vi "Fetch Trace (Reflection Measurement).vi"(8 "error in (no error)":errorcluster, 9 "Timeout (10000ms)":i32=10000, 10 "Data Type (0: Data)":i32(ring) items=["Data", "Memory"], 11 "VISA resource name":refnum<visa-resource-name>) -> (0 "error out":errorcluster, 2 "Trace Data":dbl[](array[numeric]), 3 "VISA resource name out":refnum<visa-resource-name>)   [LabVIEW 2022 SP3, in "Agilent N934X Series.lvlib"]
doc: "Fetches trace of Reflection Measurement from the spectrum analyzer and does not initiate data acquisition.\n\nNote:\n\nThis VI does not check the instrument status. Typically, you call this VI only in a sequence of calls to other low-level instrument driver VIs. The sequence performs one operation. You use the low-level VIs to optimize one or more aspects of interaction with the instrument. If you want to check the instrument status, call the <B>Error Query VI</B> at the conclusion of the sequence.\n\nThis VI is only applicable for N9321C, N9322C, N9323C, N9324C models."
uses:
  <instrlib>/Agilent N934X Series/Agilent N934X Series.lvlib
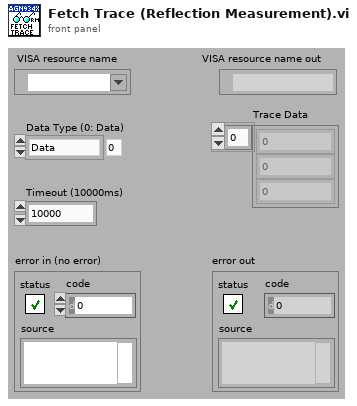
[diagram p1: front panel]
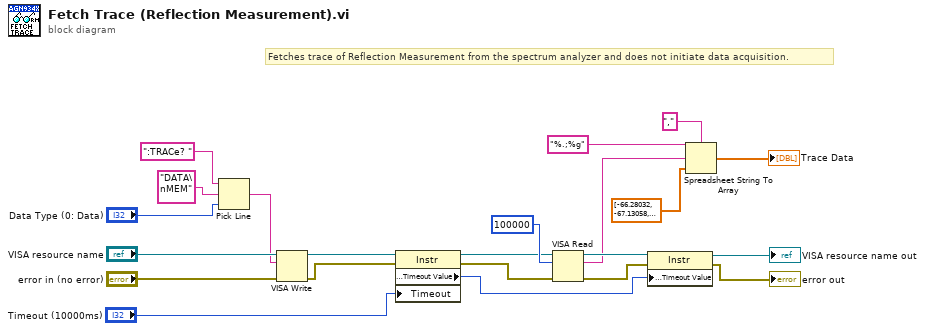
[diagram p0: block diagram]
diagram:
  # "Fetches trace of Reflection Measurement from the spectrum analyzer and does not initiate data acquisition."
  n1 = Pick Line(string ("")=":TRACe? ", multi-line string="DATA\nMEM", line index="Data Type (0: Data)") -> (output string=w2:string)
  n2 = VISA Write(VISA resource name="VISA resource name", write buffer=w2, error in (no error)="error in (no error)") -> (VISA resource name out=w19:refnum<visa-resource-name>, error out=w18:errorcluster)  [unwired: 1 out]
  n3 = property class="Instr"(reference=w19, error in=w18, "Timeout"="Timeout (10000ms)") -> (reference out=w17:refnum<visa-resource-name>, error out=w16:errorcluster, "General Settings:Timeout Value"=w14:u32)
  n4 = VISA Read(VISA resource name=w17, byte count=u32 100000, error in (no error)=w16) -> (VISA resource name out=w13:refnum<visa-resource-name>, read buffer=w11:string, error out=w12:errorcluster)  [unwired: 1 out]
  n5 = property class="Instr"(reference=w13, error in=w12, "General Settings:Timeout Value"=w14) -> (reference out=→"VISA resource name out":refnum<visa-resource-name>, error out=→"error out":errorcluster)
  n6 = Spreadsheet String To Array(delimiter (Tab)=",", format string="%.;%g", spreadsheet string=w11, array type (2D Dbl)=dbl[] [-66.28032, -67.13058, -67.71282, -69.11133, -72.48418, -68.59103, -74.18298, -67.65571, -67.90143, -68.77035, -69.91087, -65.28284, -72.02601, -68.77459, -70.57571] ("Trace Data")) -> (array=→"Trace Data":dbl[])
